vi "Connect Channels (Single).vi"(8 "error in (no error)":errorcluster, 9 "channel 2":string, 10 "channel 1":string, 11 "SLSC Switch in":refnum<class "SLSC Switch.lvclass">) -> (0 "error out":errorcluster, 3 "SLSC Switch out":refnum<class "SLSC Switch.lvclass">)   [LabVIEW 2015, in "SLSC Switch.lvclass"]
uses:
  SLSC Switch.lvclass
  SLSC Switch.lvclass/SLSC Switch.ctl
  slscsl/slscsl.lvclass
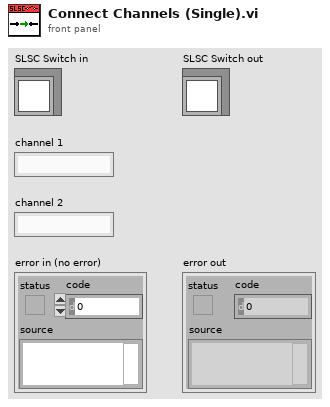
[diagram p1: front panel]
types:
  T1 = typedef "slscsl.lvclass/SwitchActionList.ctl" = T2[]
  T2 = typedef "slscsl.lvclass/SwitchAction.ctl" = cluster{"index":i32, "position":T3}
  T3 = typedef "slscsl.lvclass/RelayPosition.ctl" = i32
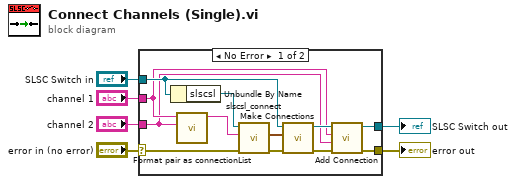
[diagram p0: block diagram]
diagram:
  n1 = case shown="No Error" "error in (no error)" {
    selector: "error in (no error)" -> [w15 w20]
    tunnel: [w9 w20] -> w5
    tunnel: [w10 w19] -> w3
    tunnel: "SLSC Switch in" -> [w13 w19]
    tunnel: "channel 1" -> [w8 _]
    tunnel: "channel 2" -> [w7 _]
    frame No Error {
      n2 = Unbundle By Name(w13) -> ("slscsl"=w16:refnum<class "slscsl.lvclass">)
      n3 = call "Format pair as connectionList.vi"("channel in"=w7, "channel 1"=w8) -> ("connectionList"=w14:string)  [unwired: 9 in]
      n4 = call "slscsl_connect.vi"("error in (no error)"=w15, "connectionList"=w14, "Route Manager in"=w16) -> ("error out"=w17:errorcluster, "SwitchActionList"=w18:T1)  [unwired: 6 in, 1 out]
      n5 = call "Make Connections.vi"("error in (no error)"=w17, "relays to open"=w18, "SLSC Switch in"=w13) -> ("error out"=w12:errorcluster, "SLSC Switch out"=w11:refnum<class "SLSC Switch.lvclass">)  [unwired: 7 in]
      n6 = call "Add Connection.vi"("error in (no error)"=w12, "channel 2"=w7, "channel 1"=w8, "SLSC Switch in"=w11) -> ("error out"=w9:errorcluster, "SLSC Switch out"=w10:refnum<class "SLSC Switch.lvclass">)  [unwired: 6 in]
    }
    frame Error {
    }
  }
  "error out" <- w5
  "SLSC Switch out" <- w3
